vi "Get All Control Ref.vi"(11 "reference":refnum<vi>) -> (1 "String 2":string, 2 "Output Array":string[](array[string]), 3 "Controls[]":refnum<vi>[](array[refnum]))   [LabVIEW 2021]
panel:
  out "size(s) 2":i32
  out "size(s)":i32
  out "Array":string[](array[string])
  in  "Outer Cluster":T1 {"Horizontal" scale=0.0..10.0}
  in  "OK Button":bool
  in  "String":string
  in  "Tab Control":enum32{"Page 1", "Page 2"}(tab)
  in  "Array List":i32[](array[listbox])
  in  "Numeric":dbl
  in  "Inner Cluster":T2 {"Vertical" scale=0.0..10.0}
  in  "Boolean":bool
  # "Overview: This example demonstrates how to list all object on the front panel\nRequirement: NI LabVIEW 12.0 or compatible\nInstruction:\n1. Run the VI"
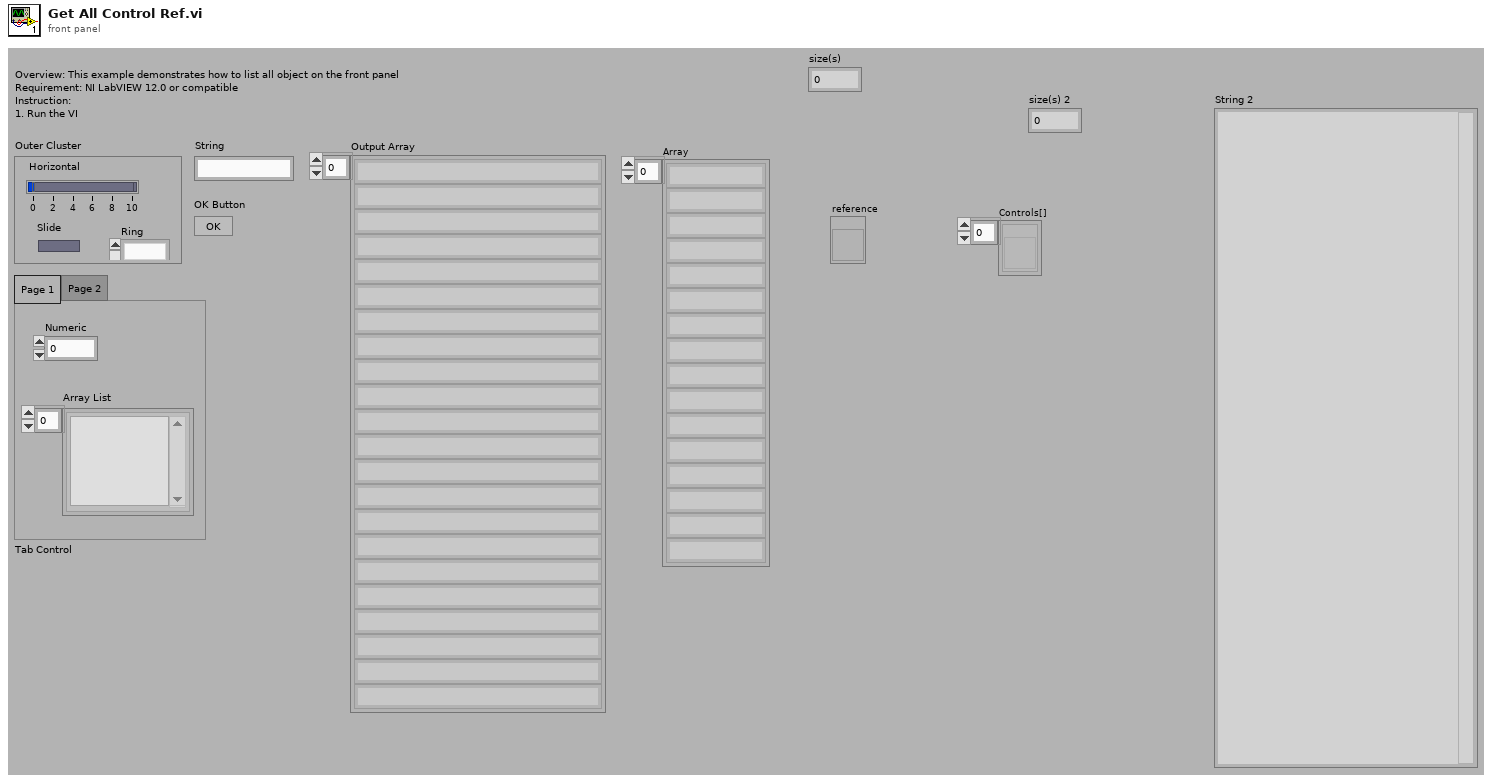
[diagram p1: front panel]
types:
  T1 = cluster{"Horizontal":dbl, "Slide":bool, "Ring":u16}
  T2 = cluster{"Vertical":dbl, "Toggle":bool, "Enum":enum16{""}}
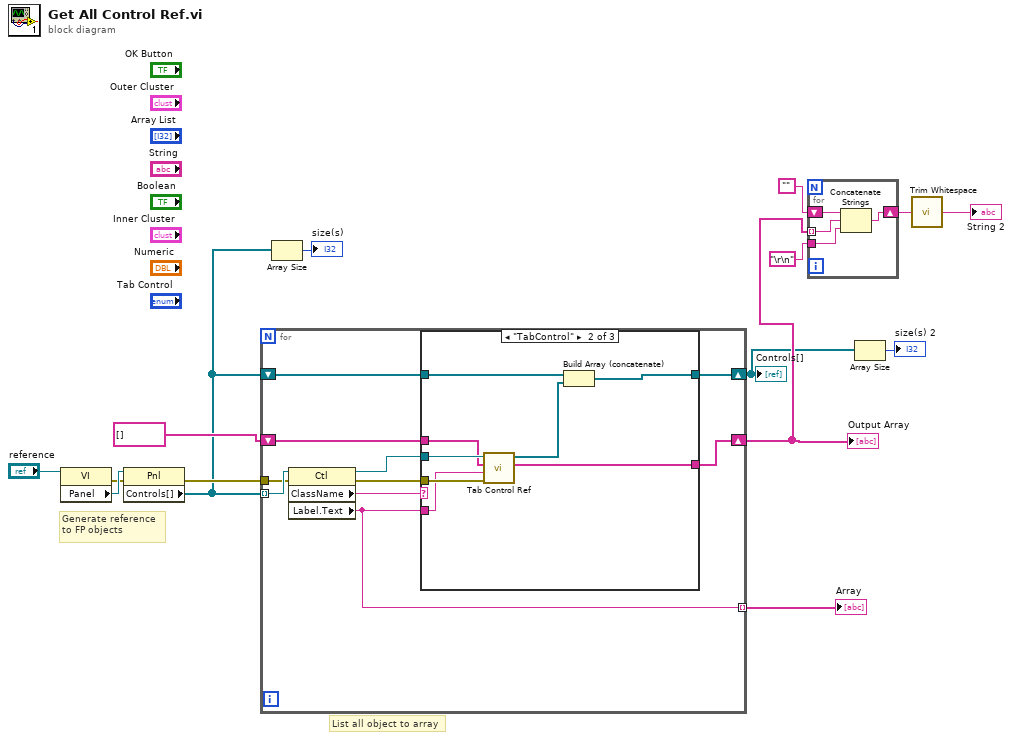
[diagram p0: block diagram]
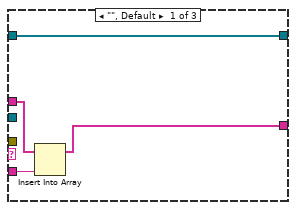
[diagram p2: hidden frame]
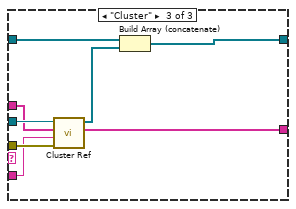
[diagram p3: hidden frame]
diagram:
  # "List all object to array"
  # "Generate reference \nto FP objects"
  n1 = property class="VI"(reference="reference") -> (error out=w14:errorcluster, "Panel"=w15:refnum<vi>)  [unwired: 1 in, 1 out]
  n2 = property class="Pnl"(reference=w15, error in=w14) -> (error out=w13:errorcluster, "Controls[]"=w4:refnum<vi>[])  [unwired: 1 out]
  n3 = for {
    tunnel: w4 -> [w25] mode=indexing
    tunnel: w13 -> [w24]
    shift-right: [w20] -> w5
    shift-left: string[] [] ("Array") -> [w19]
    tunnel: [w18] -> w11 mode=indexing
    shift-right: [w17] -> w1
    shift-left: w4 -> [w16]
    n4 = property class="Ctl"(reference=w25, error in=w24) -> (reference out=w22:refnum<vi>, error out=w21:errorcluster, "ClassName"=w23:string, "Label.Text"=w18:string)
    n5 = case shown="\"TabControl\"" w23 {
      tunnel: w22 -> [_ w37 w45]
      tunnel: w21 -> [_ w36 w44]
      tunnel: [w28 w34 w41] -> w20
      tunnel: w19 -> [w29 w35 w43]
      tunnel: w18 -> [w27 w33 w42]
      tunnel: [w26 w31 w39] -> w17
      tunnel: w16 -> [w26 w32 w40]
      frame "", Default {
        n6 = Insert Into Array(array=w29, new element=w27) -> (w28:string[])  [unwired: 1 in]
      }
      frame "TabControl" {
        n7 = call "Tab Control Ref.vi"("error out"=w36, "Label Text"=w33, "Array In"=w35, "TabControl Reference"=w37) -> ("Array Out"=w34:string[], "ControlsOnPage"=w30:refnum<vi>[])  [unwired: 6 in]
        n8 = Build Array (concatenate)(w32, w30) -> (w31:refnum<vi>[])
      }
      frame "Cluster" {
        n9 = call "Cluster Ref.vi"("error out"=w44, "Label Text"=w42, "Input Array"=w43, "Cluster Reference"=w45) -> ("Array Out"=w41:string[], "Controls[]"=w38:refnum<vi>[])  [unwired: 6 in]
        n10 = Build Array (concatenate)(w40, w38) -> (w39:refnum<vi>[])
      }
    }
  }
  "Output Array" <- w5
  "Array" <- w11
  "Controls[]" <- w1
  n11 = Array Size(array=w4) -> (size(s)=→"size(s)":i32)
  n12 = for {
    tunnel: w5 -> [w48] mode=indexing
    shift-right: [w46] -> w8
    shift-left: "" -> [w49]
    tunnel: "\r\n" -> [w47]
    n13 = Concatenate Strings(w49, w48, w47) -> (w46:string)
  }
  n14 = Array Size(array=w1) -> (size(s)=→"size(s) 2":i32)
  n15 = call <vilib>:"Trim Whitespace.vi"("string"=w8) -> ("trimmed string"=→"String 2":string)  [unwired: 1 in]
